vi "Digest Banana.vi"(8 "error in":errorcluster, 11 "Platano":refnum<class "Platano.lvclass">) -> (0 "error out":errorcluster)   [LabVIEW 2021, in "Bananas.lvlib"]
uses:
  Bananas.lvlib
  Banana/Banana.lvclass
  Banana Core Actions -- enum.ctl
  Platano/Platano.lvclass
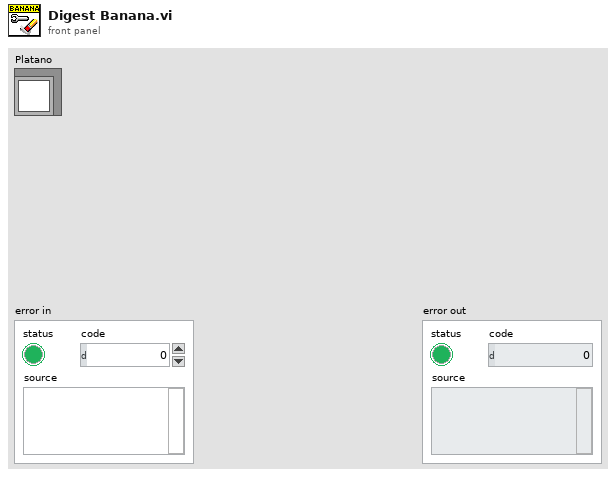
[diagram p1: front panel]
types:
  T1 = typedef "Bananas.lvlib/Platano.lvclass/Banana Core Actions -- enum.ctl" = enum16{"Get/Set", "Clear", "Discard"}
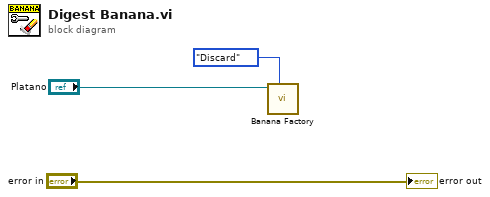
[diagram p0: block diagram]
diagram:
  n1 = call "Banana Factory.vi"("Action"=Banana_Core_Actions_--_enum."Discard", "Platano"="Platano") -> ()  [unwired: 9 in, 1 out]
  "error out" <- "error in"
